vi "Update Queue Nested.vi"(9 "Insert (T) or Remove (F)":bool, 10 "Queue Nested":map{string, refnum<data-value>}(c390), 11 "Base Event jettl in":refnum<class "Base Event jettl.lvclass">) -> (3 "Base Event jettl out":refnum<class "Base Event jettl.lvclass">)   [LabVIEW 2021, in "jettl.lvlib" / "Base Event jettl.lvlib" / "Base Event jettl.lvclass"]
uses:
  Base Event jettl.lvclass
  Msg Strategy/Msg Strategy/Msg Strategy.lvclass
  Base Event jettl.lvclass/Base Event jettl.ctl
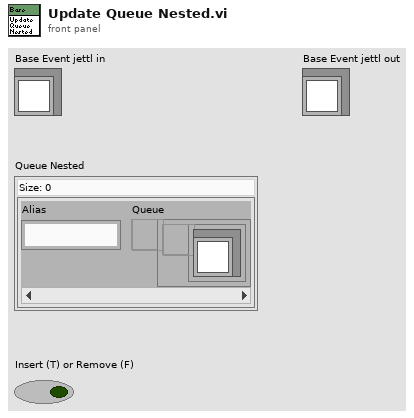
[diagram p1: front panel]
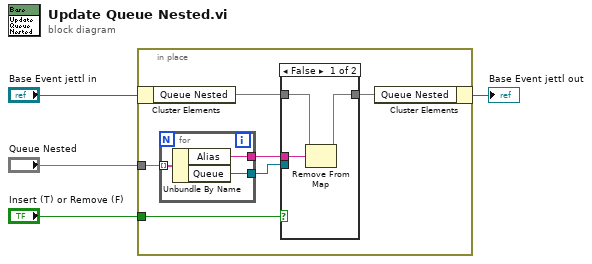
[diagram p0: block diagram]
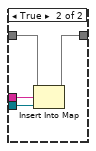
[diagram p2: hidden frame]
diagram:
  n1 = in-place {
    in-place-border: "Queue Nested" -> [w8]
    in-place-border: "Insert (T) or Remove (F)" -> [w5]
    n2 = in-place-cluster #1("Base Event jettl in") -> ("Queue Nested"=w10:map{string, refnum<data-value>})
    n3 = for {
      tunnel: w8 -> [w20] mode=indexing
      tunnel: [w19] -> w7
      tunnel: [w18] -> w6
      n4 = Unbundle By Name(w20) -> ("Alias"=w19:string, "Queue"=w18:refnum<data-value>)
    }
    n5 = case shown="False" w5 {
      tunnel: w10 -> [w13 w17]
      tunnel: [w12 w16] -> w9
      tunnel: w7 -> [w11 w15]
      tunnel: w6 -> [_ w14]
      frame False {
        n6 = Remove From Map(10:w11, 11:w13) -> (3:w12:map{string, refnum<data-value>})  [unwired: 2 out]
      }
      frame True {
        n7 = Insert Into Map(map in=w17, key=w15, value=w14) -> (map out=w16:map{string, refnum<data-value>})  [unwired: 2 out]
      }
    }
    n8 = in-place-cluster #1("Queue Nested"=w9) -> (→"Base Event jettl out":refnum<class "Base Event jettl.lvclass">)
  }
